vi "LVClass_WavefrontCorrector Get parameters whose differ from WavefrontCorrectorSet.vi"(0 "WavefrontCorrector in":refnum<class "WavefrontCorrector.lvclass">, 5 "WavefrontCorrectorSet in":refnum<class "WavefrontCorrectorSet.lvclass">, 11 "error in (no error)":errorcluster) -> (4 "WavefrontCorrector out":refnum<class "WavefrontCorrector.lvclass">, 6 "WavefrontCorrectorSet out":refnum<class "WavefrontCorrectorSet.lvclass">, 12 "nb_nonequals_settable_connection_params":i32, 13 "nb_nonequals_onfly_settable_params":i32, 14 "nb_nonequal_settable_params":i32, 15 "error out":errorcluster)   [LabVIEW 2020, in "WavefrontCorrector.lvclass"]
doc: "Wavefront corrector parameter getter for parameter of type boolean.\n\n--------------------------------------------------------------------------------\n\n<B>correctorIn </B> : WavefrontCorrector object.\n<B>correctorOut </B> : WavefrontCorrector object.\n<B>parameter_name </B> : Name of the parameter.\n<B>value </B> : Value of the parameter.\n<B>ErrorIn </B> : Error\n<B>ErrorOut </B> : Error\n\n--------------------------------------------------------------------------------"
uses:
  WavefrontCorrector.lvclass
  WavefrontCorrectorSet/WavefrontCorrectorSet.lvclass
  WavefrontCorrector.lvclass/WavefrontCorrector.ctl
  WavefrontCorrectorSet/LVClass_WavefrontCorrectorSet Read WavefrontCorrectorSet.vi
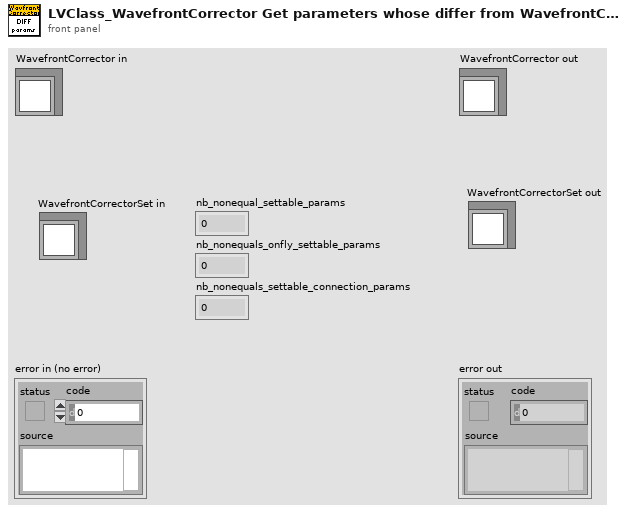
[diagram p1: front panel]
types:
  T1 = typedef "ClassID.ctl" = i64
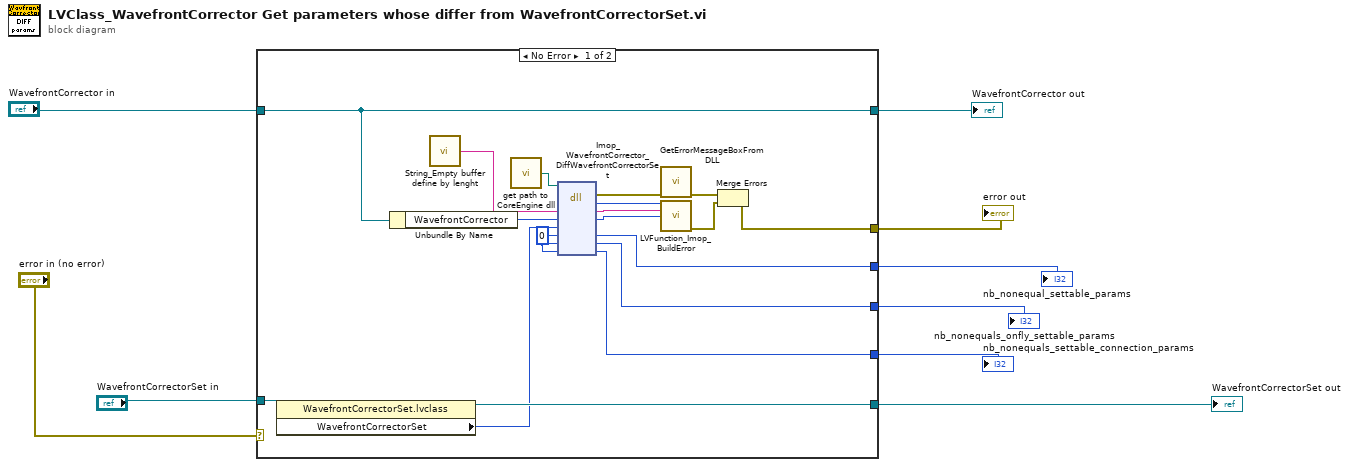
[diagram p0: block diagram]
diagram:
  n1 = case shown="No Error" "error in (no error)" {
    selector: "error in (no error)" -> [_ w29]
    tunnel: [w16 w29] -> w5
    tunnel: [w26 w28] -> w4
    tunnel: "WavefrontCorrector in" -> [w26 w28]
    tunnel: [w17 _] -> w7
    tunnel: "WavefrontCorrectorSet in" -> [w18 _]
    tunnel: [w14 _] -> w3
    tunnel: [w13 _] -> w2
    tunnel: [w12 _] -> w1
    frame No Error {
      w11 = 0 ("nb_nonequal_settable_params")
      n2 = property class="WavefrontCorrectorSet.lvclass"(reference=w18) -> (reference out=w17:refnum<class "WavefrontCorrectorSet.lvclass">, "WavefrontCorrectorSet"=w15:T1)  [unwired: 1 in, 1 out]
      n3 = Unbundle By Name(w26) -> ("WavefrontCorrector"=w25:T1)
      n4 = call "String_Empty buffer define by lenght.vi"() -> ("Empty buffer"=w27:string)  [unwired: 1 in]
      n5 = call "get path to CoreEngine dll.vi"() -> ("path to wavekit library"=w22:path)  [unwired: 14 in, 1 out]
      n6 = dll-call lib="D:/soft/HASO_v3/SVN_trunk/ImOpCoreEngine4_LV2011/DLLs/c_interface_vc100.dll" fn="Imop_WavefrontCorrector_DiffWavefrontCorrectorSet"(path in=w22, "message"=w27, "camera"=w25, "CameraSet"=w15, "nb_nonequal_settable_params"=w11, "nb_nonequals_onfly_settable_params"=w11, "nb_nonequals_settable_connection_params"=w11) -> (error out=w21:errorcluster, "return type"=w23:i32, "message"=w24:string, "camera"=w10:i64, "nb_nonequal_settable_params"=w14:i32, "nb_nonequals_onfly_settable_params"=w13:i32, "nb_nonequals_settable_connection_params"=w12:i32)  [unwired: 3 in, 1 out]
      n7 = call "GetErrorMessageBoxFromDLL.vi"("error IN"=w21) -> ("error OUT"=w20:errorcluster)  [unwired: 10 in]
      n8 = call "LVFunction_Imop_BuildError.vi"("code"=w23, "String to Prepend to source (\"\")"=w24, "Adresse"=w10) -> ("error out"=w19:errorcluster)  [unwired: 12 in]
      n9 = Merge Errors(w20, w19) -> (w16:errorcluster)
    }
    frame Error {
    }
  }
  "error out" <- w5
  "WavefrontCorrector out" <- w4
  "WavefrontCorrectorSet out" <- w7
  "nb_nonequal_settable_params" <- w3
  "nb_nonequals_onfly_settable_params" <- w2
  "nb_nonequals_settable_connection_params" <- w1
